vi "readAllSettings.vi"(8 "error in (no error)":errorcluster) -> (0 "error out":errorcluster, 3 "ILC Settings":T1={"Collection Settings"={"Samples To Average"=1, "Test Delay"=0.01}, "TestExecutionOrder"=[], "Verify Voltage Tests"={"+3.3VD"={"DAQ Channel to Read"="ai3", "Expected Value"=0.0, "Tolerance"=0.0}, "+5.1V"={"DAQ Channel to Read"="ai3", "Expected Value"=0.0, "Tolerance"=0.0}, "RELVALV1"={"DAQ Channel to Read"="", "Expected Value"=0.0, "Tolerance"=0.0}, "RELVALV2"={"DAQ Channel to Read"="", "Expected Value"=0.0, "Tolerance"=0.0}}, "Verify DAC Tests"={"DAC A Channels"={"DAQ Channel 1 to Read"="ai5", "DAQ Channel 2 to Read"="ai6", "Resistor Ohms"=0.0}, "DAC B Channels"={"DAQ Channel 1 to Read"="ai7", "DAQ Channel 2 to Read"="ai8", "Resistor Ohms"=0.0}, "DAC = -1.00A"={"Expected Value"=-1.0, "Tolerance"=0.001}, "DAC = -0.75A"={"Expected Value"=-0.75, "Tolerance"=0.00075}, "DAC = -0.50A"={"Expected Value"=-0.5, "Tolerance"=0.0005}, "DAC = -0.25A"={"Expected Value"=-0.25, "Tolerance"=0.00025}, "DAC = 0.00A"={"Expected Value"=0.0, "Tolerance"=0.0001}, "DAC = 0.25A"={"Expected Value"=0.25, "Tolerance"=0.00025}, "DAC = 0.50A"={"Expected Value"=0.5, "Tolerance"=0.0005}, "DAC = 0.75A"={"Expected Value"=0.75, "Tolerance"=0.00075}, "DAC = 1.00A"={"Expected Value"=1.0, "Tolerance"=0.001}}, "Set DAC Tests"={"DAC = 0.00A"={"Command Value"=34224}, "DAC = 0.25A"={"Command Value"=42052}, "DAC = 0.5A"={"Command Value"=49879}, "DAC = 0.75A"={"Command Value"=57707}, "DAC = 1.0A"={"Command Value"=65535}, "DAC = -0.25A"={"Command Value"=26396}, "DAC = -0.5A"={"Command Value"=18568}, "DAC = -0.75A"={"Command Value"=10740}, "DAC = -1.0A"={"Command Value"=0}}, "Enable Disable"={"Motor Enable"=255, "Motor Disable"=0, "Current Output Enable"=1, "Current Output Disable"=0, "Power Enable"=0, "Power Disable"=1, "Amplifier Enable"=0, "Amplifier Disable"=1}, "Pressure Tests"={"0% Test"={"Command"=0, "Expected"=1933, "Tolerance"=492}, "25% Test"={"Command"=12322, "Expected"=4095, "Tolerance"=492}, "50% Test"={"Command"=26326, "Expected"=6553, "Tolerance"=492}, "75% Test"={"Command"=40329, "Expected"=9010, "Tolerance"=492}, "100% Test"={"Command"=54332, "Expected"=11468, "Tolerance"=492}, "Settling (ms)"=500, "Delay (ms)"=10}} {"Verify DAC Tests"."DAC = 1.00A"."Tolerance" format="%.6f"; "Verify DAC Tests"."DAC = 1.00A"."Expected Value" format="%.3f"; "Verify DAC Tests"."DAC = 0.75A"."Tolerance" format="%.6f"; "Verify DAC Tests"."DAC = 0.75A"."Expected Value" format="%.3f"; "Verify DAC Tests"."DAC = 0.50A"."Tolerance" format="%.6f"; "Verify DAC Tests"."DAC = 0.50A"."Expected Value" format="%.3f"; "Verify DAC Tests"."DAC = 0.25A"."Tolerance" format="%.6f"; "Verify DAC Tests"."DAC = 0.25A"."Expected Value" format="%.3f"; "Verify DAC Tests"."DAC = 0.00A"."Tolerance" format="%.6f"; "Verify DAC Tests"."DAC = 0.00A"."Expected Value" format="%.3f"; "Verify DAC Tests"."DAC = -0.25A"."Tolerance" format="%.6f"; "Verify DAC Tests"."DAC = -0.25A"."Expected Value" format="%.3f"; "Verify DAC Tests"."DAC = -0.50A"."Tolerance" format="%.6f"; "Verify DAC Tests"."DAC = -0.50A"."Expected Value" format="%.3f"; "Verify DAC Tests"."DAC = -0.75A"."Tolerance" format="%.6f"; "Verify DAC Tests"."DAC = -0.75A"."Expected Value" format="%.3f"; "Verify DAC Tests"."DAC = -1.00A"."Tolerance" format="%.6f"; "Verify DAC Tests"."DAC = -1.00A"."Expected Value" format="%.3f"; "Verify DAC Tests"."DAC B Channels"."Resistor Ohms" format="%.3g"; "Verify DAC Tests"."DAC A Channels"."Resistor Ohms" format="%.3g"; "Verify Voltage Tests"."RELVALV2"."Tolerance" format="%.6f"; "Verify Voltage Tests"."RELVALV2"."Expected Value" format="%.3f"; "Verify Voltage Tests"."RELVALV1"."Tolerance" format="%.6f"; "Verify Voltage Tests"."RELVALV1"."Expected Value" format="%.3f"; "Verify Voltage Tests"."+5.1V"."Tolerance" format="%.6f"; "Verify Voltage Tests"."+5.1V"."Expected Value" format="%.3f"; "Verify Voltage Tests"."+3.3VD"."Tolerance" format="%.6f"; "Verify Voltage Tests"."+3.3VD"."Expected Value" format="%.3f"})   [LabVIEW 2015]
uses:
  Typedefs/Test Settings.ctl
  Typedefs/Collection Settings.ctl
  Typedefs/TestExecutionOrder.ctl
  Typedefs/TestScenarioTypes.ctl
  Typedefs/Verify Voltage Tests.ctl
  Typedefs/Verify Voltage Test.ctl
  Typedefs/Verify DAC Tests.ctl
  Typedefs/DAC Channels.ctl
  Typedefs/Verify DAC Test.ctl
  Typedefs/Set DAC Tests.ctl
  Typedefs/Set DAC Test.ctl
  Typedefs/Enable Disable.ctl
  Typedefs/Pressure Tests.ctl
  Typedefs/Pressure Test.ctl
  ConfigurationTestParameters/ConfigurationTestParameters.lvclass
  Typedefs/ILCBTTypedefs.lvlib
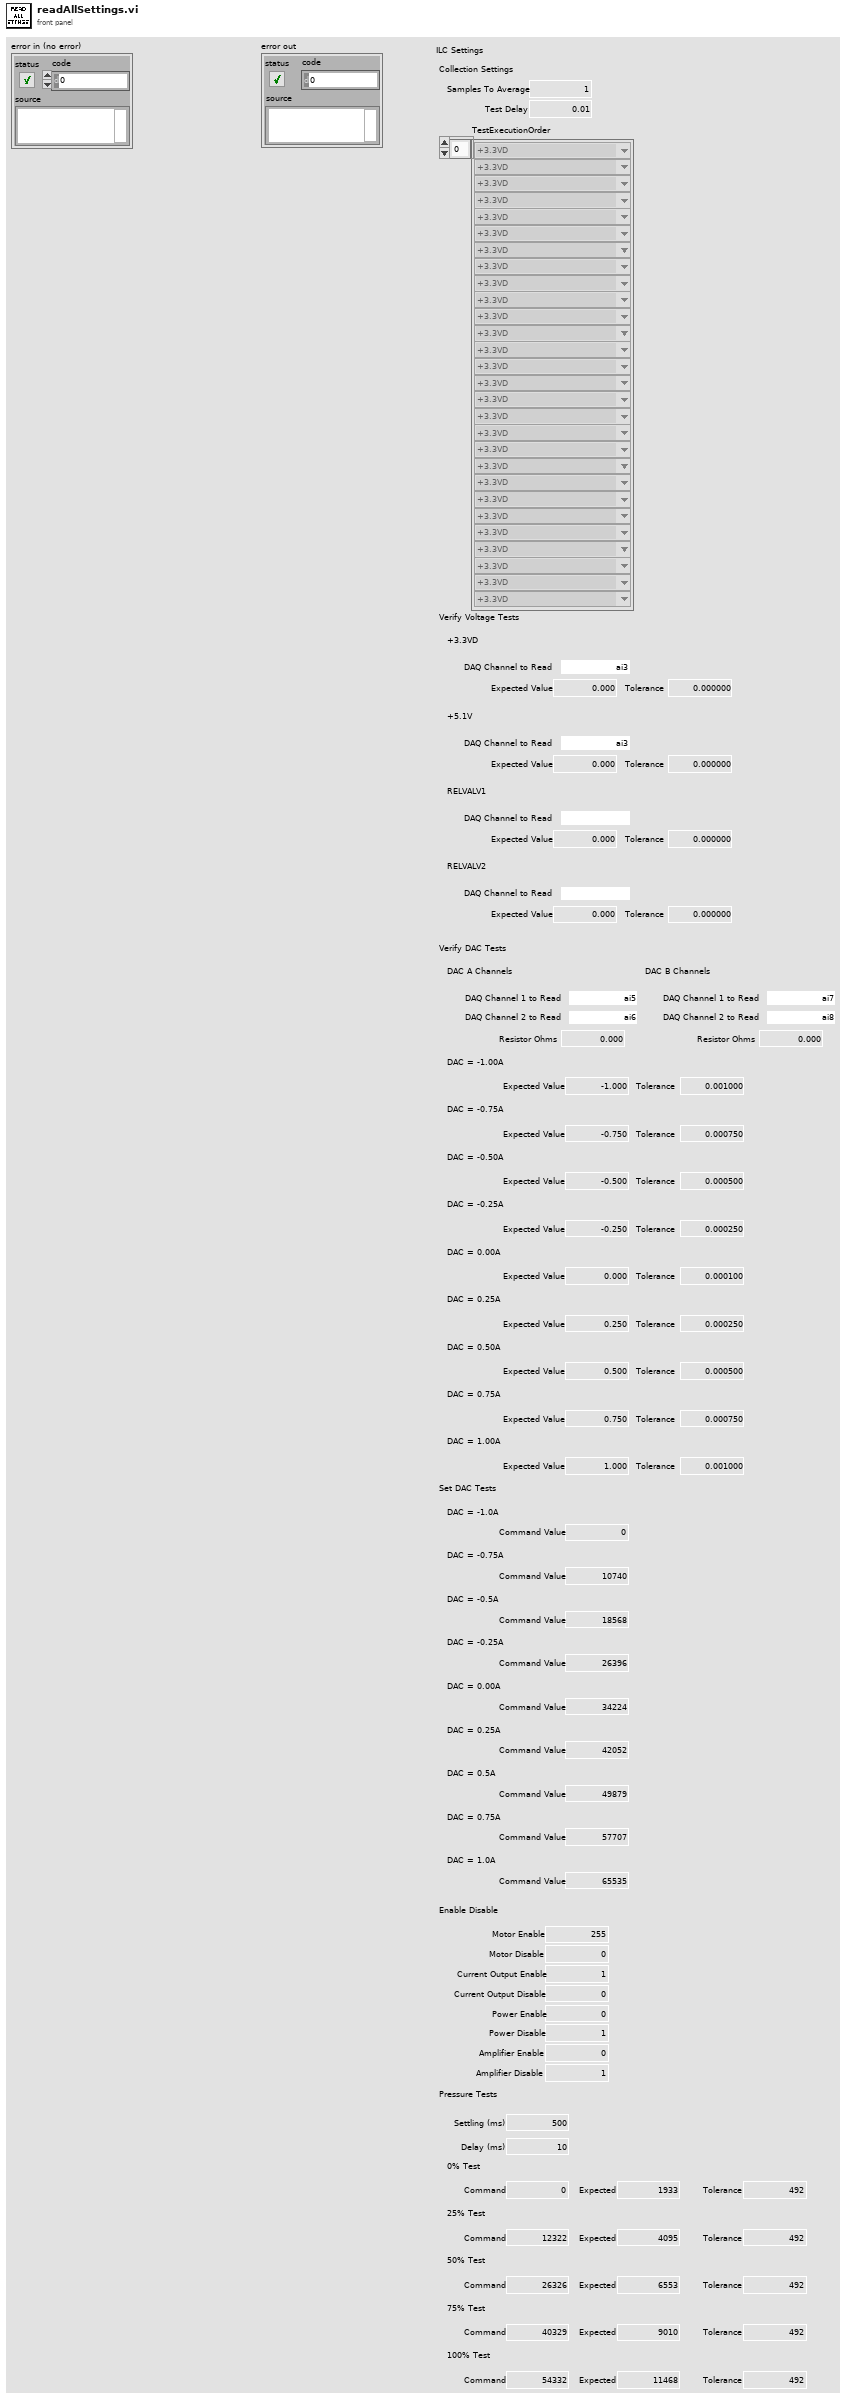
[diagram p1: front panel]
types:
  T1 = typedef "ILCBTTypedefs.lvlib/Test Settings.ctl" = cluster{"Collection Settings":T2, "TestExecutionOrder":T3, "Verify Voltage Tests":T5, "Verify DAC Tests":T7, "Set DAC Tests":T10, "Enable Disable":T12, "Pressure Tests":T13}
  T2 = typedef "ILCBTTypedefs.lvlib/Collection Settings.ctl" = cluster{"Samples To Average":i32, "Test Delay":dbl}
  T3 = typedef "ILCBTTypedefs.lvlib/TestExecutionOrder.ctl" = T4[]
  T4 = typedef "ILCBTTypedefs.lvlib/TestScenarioTypes.ctl" = enum16{"+3.3VD", "+5.1V", "+24V", "RELVALV1", "RELVALV2", "Verify DAC_A = -1.00A", "Verify DAC_A = -0.75A", "Verify DAC_A = -0.50A", "Verify DAC_A = -0.25A", "Verify DAC_A = 0.00A", "Verify DAC_A = 0.25A", "Verify DAC_A = 0.50A", "Verify DAC_A = 0.75A", "Verify DAC_A = 1.00A", "Verify DAC_B = -1.00A", "Verify DAC_B = -0.75A", "Verify DAC_B = -0.50A", "Verify DAC_B = -0.25A", "Verify DAC_B = 0.00A", "Verify DAC_B = 0.25A", "Verify DAC_B = 0.50A", "Verify DAC_B = 0.75A", "Verify DAC_B = 1.00A", "Set DAC_A = -1.00A", "Set DAC_A = -0.75A", "Set DAC_A = -0.50A", "Set DAC_A = -0.25A", "Set DAC_A = 0.00A", "Set DAC_A = 0.25A", "Set DAC_A = 0.50A", "Set DAC_A = 0.75A", "Set DAC_A = 1.00A", "Set DAC_B = -1.00A", "Set DAC_B = -0.75A", "Set DAC_B = -0.50A", "Set DAC_B = -0.25A", "Set DAC_B = 0.00A", "Set DAC_B = 0.25A", "Set DAC_B = 0.50A", "Set DAC_B = 0.75A", "Set DAC_B = 1.00A", "Set MTR_PWR = On", "Set MTR_PWR = Off", "Set OUTPUT = On", "Set OUTPUT = Off", "Verify OUTPUT = On", "Verify OUTPUT = Off", "Verify POWER = Ok", "Verify POWER = Fail", "Verify AMP1 = Ok", "Verify AMP1 = Fail", "Verify AMP2 = Ok", "Verify AMP2 = Fail", "P1 0%", "P1 25%", "P1 50%", "P1 75%", "P1 100%", "P2 0%", "P2 25%", "P2 50%", "P2 75%", "P2 100%", "P3 0%", "P3 25%", "P3 50%", "P3 75%", "P3 100%", "P4 0%", "P4 25%", "P4 50%", "P4 75%", "P4 100%"}
  T5 = typedef "ILCBTTypedefs.lvlib/Verify Voltage Tests.ctl" = cluster{"+3.3VD":T6, "+5.1V":T6, "RELVALV1":T6, "RELVALV2":T6}
  T6 = typedef "ILCBTTypedefs.lvlib/Verify Voltage Test.ctl" = cluster{"DAQ Channel to Read":refnum<k21>, "Expected Value":dbl, "Tolerance":dbl}
  T7 = typedef "ILCBTTypedefs.lvlib/Verify DAC Tests.ctl" = cluster{"DAC A Channels":T8, "DAC B Channels":T8, "DAC = -1.00A":T9, "DAC = -0.75A":T9, "DAC = -0.50A":T9, "DAC = -0.25A":T9, "DAC = 0.00A":T9, "DAC = 0.25A":T9, "DAC = 0.50A":T9, "DAC = 0.75A":T9, "DAC = 1.00A":T9}
  T8 = typedef "ILCBTTypedefs.lvlib/DAC Channels.ctl" = cluster{"DAQ Channel 1 to Read":refnum<k21>, "DAQ Channel 2 to Read":refnum<k21>, "Resistor Ohms":dbl}
  T9 = typedef "ILCBTTypedefs.lvlib/Verify DAC Test.ctl" = cluster{"Expected Value":dbl, "Tolerance":dbl}
  T10 = typedef "ILCBTTypedefs.lvlib/Set DAC Tests.ctl" = cluster{"DAC = 0.00A":T11, "DAC = 0.25A":T11, "DAC = 0.5A":T11, "DAC = 0.75A":T11, "DAC = 1.0A":T11, "DAC = -0.25A":T11, "DAC = -0.5A":T11, "DAC = -0.75A":T11, "DAC = -1.0A":T11}
  T11 = typedef "ILCBTTypedefs.lvlib/Set DAC Test.ctl" = cluster{"Command Value":u16}
  T12 = typedef "ILCBTTypedefs.lvlib/Enable Disable.ctl" = cluster{"Motor Enable":u16, "Motor Disable":u16, "Current Output Enable":u16, "Current Output Disable":u16, "Power Enable":u16, "Power Disable":u16, "Amplifier Enable":u16, "Amplifier Disable":u16}
  T13 = typedef "ILCBTTypedefs.lvlib/Pressure Tests.ctl" = cluster{"0% Test":T14, "25% Test":T14, "50% Test":T14, "75% Test":T14, "100% Test":T14, "Settling (ms)":u16, "Delay (ms)":u16}
  T14 = typedef "ILCBTTypedefs.lvlib/Pressure Test.ctl" = cluster{"Command":u16, "Expected":u16, "Tolerance":u16}
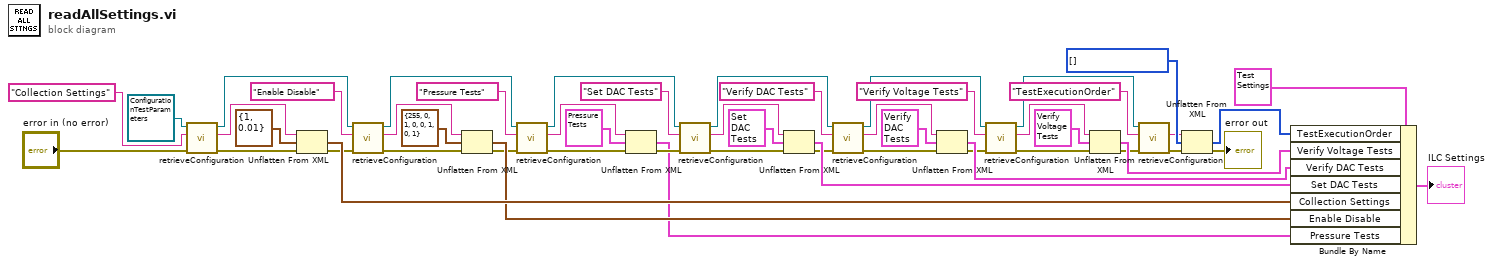
[diagram p0: block diagram]
diagram:
  w24 = T3 [] items=["+3.3VD", "+5.1V", "+24V", "RELVALV1", "RELVALV2", "Verify DAC_A = -1.00A", "Verify DAC_A = -0.75A", "Verify DAC_A = -0.50A", "Verify DAC_A = -0.25A", "Verify DAC_A = 0.00A", "Verify DAC_A = 0.25A", "Verify DAC_A = 0.50A", "Verify DAC_A = 0.75A", "Verify DAC_A = 1.00A", "Verify DAC_B = -1.00A", "Verify DAC_B = -0.75A", "Verify DAC_B = -0.50A", "Verify DAC_B = -0.25A", "Verify DAC_B = 0.00A", "Verify DAC_B = 0.25A", "Verify DAC_B = 0.50A", "Verify DAC_B = 0.75A", "Verify DAC_B = 1.00A", "Set DAC_A = -1.00A", "Set DAC_A = -0.75A", "Set DAC_A = -0.50A", "Set DAC_A = -0.25A", "Set DAC_A = 0.00A", "Set DAC_A = 0.25A", "Set DAC_A = 0.50A", "Set DAC_A = 0.75A", "Set DAC_A = 1.00A", "Set DAC_B = -1.00A", "Set DAC_B = -0.75A", "Set DAC_B = -0.50A", "Set DAC_B = -0.25A", "Set DAC_B = 0.00A", "Set DAC_B = 0.25A", "Set DAC_B = 0.50A", "Set DAC_B = 0.75A", "Set DAC_B = 1.00A", "Set MTR_PWR = On", "Set MTR_PWR = Off", "Set OUTPUT = On", "Set OUTPUT = Off", "Verify OUTPUT = On", "Verify OUTPUT = Off", "Verify POWER = Ok", "Verify POWER = Fail", "Verify AMP1 = Ok", "Verify AMP1 = Fail", "Verify AMP2 = Ok", "Verify AMP2 = Fail", "P1 0%", "P1 25%", "P1 50%", "P1 75%", "P1 100%", "P2 0%", "P2 25%", "P2 50%", "P2 75%", "P2 100%", "P3 0%", "P3 25%", "P3 50%", "P3 75%", "P3 100%", "P4 0%", "P4 25%", "P4 50%", "P4 75%", "P4 100%"] ("TestExecutionOrder")
  n1 = call "retrieveConfiguration.vi"("error in (no error)"="error in (no error)", "configName"="Collection Settings", "ConfigurationThisComponent in"=refnum<class "ConfigurationTestParameters.lvclass"> refnum ("ConfigurationTestParameters.lvclass")) -> ("error out"=w18:errorcluster, "xmlConfig"=w17:string, "ConfigurationThisComponent out"=w16:refnum<class "ConfigurationTestParameters.lvclass">)  [unwired: 6 in]
  n2 = Unflatten From XML(xml string=w17, type=T2 {"Samples To Average"=1, "Test Delay"=0.01} ("Collection Settings"), error in (no error)=w18) -> (value=w52:T2, error out=w15:errorcluster)
  n3 = call "retrieveConfiguration.vi"("error in (no error)"=w15, "configName"="Enable Disable", "ConfigurationThisComponent in"=w16) -> ("error out"=w12:errorcluster, "xmlConfig"=w13:string, "ConfigurationThisComponent out"=w6:refnum<class "ConfigurationTestParameters.lvclass">)  [unwired: 6 in]
  n4 = Unflatten From XML(xml string=w13, type=T12 {"Motor Enable"=255, "Motor Disable"=0, "Current Output Enable"=1, "Current Output Disable"=0, "Power Enable"=0, "Power Disable"=1, "Amplifier Enable"=0, "Amplifier Disable"=1} ("Enable / Disable"), error in (no error)=w12) -> (value=w10:T12, error out=w2:errorcluster)
  n5 = call "retrieveConfiguration.vi"("error in (no error)"=w2, "configName"="Pressure Tests", "ConfigurationThisComponent in"=w6) -> ("error out"=w3:errorcluster, "xmlConfig"=w4:string, "ConfigurationThisComponent out"=w5:refnum<class "ConfigurationTestParameters.lvclass">)  [unwired: 6 in]
  n6 = Unflatten From XML(xml string=w4, type=T13 {"0% Test"={"Command"=0, "Expected"=1933, "Tolerance"=492}, "25% Test"={"Command"=12322, "Expected"=4095, "Tolerance"=492}, "50% Test"={"Command"=26326, "Expected"=6553, "Tolerance"=492}, "75% Test"={"Command"=40329, "Expected"=9010, "Tolerance"=492}, "100% Test"={"Command"=54332, "Expected"=11468, "Tolerance"=492}, "Settling (ms)"=500, "Delay (ms)"=10} ("Pressure Tests"), error in (no error)=w3) -> (value=w7:T13, error out=w8:errorcluster)
  n7 = call "retrieveConfiguration.vi"("error in (no error)"=w8, "configName"="Set DAC Tests", "ConfigurationThisComponent in"=w5) -> ("error out"=w44:errorcluster, "xmlConfig"=w37:string, "ConfigurationThisComponent out"=w30:refnum<class "ConfigurationTestParameters.lvclass">)  [unwired: 6 in]
  n8 = Unflatten From XML(xml string=w37, type=T10 {"DAC = 0.00A"={"Command Value"=34224}, "DAC = 0.25A"={"Command Value"=42052}, "DAC = 0.5A"={"Command Value"=49879}, "DAC = 0.75A"={"Command Value"=57707}, "DAC = 1.0A"={"Command Value"=65535}, "DAC = -0.25A"={"Command Value"=26396}, "DAC = -0.5A"={"Command Value"=18568}, "DAC = -0.75A"={"Command Value"=10740}, "DAC = -1.0A"={"Command Value"=0}} ("Set DAC Tests"), error in (no error)=w44) -> (value=w51:T10, error out=w40:errorcluster)
  n9 = call "retrieveConfiguration.vi"("error in (no error)"=w40, "configName"="Verify DAC Tests", "ConfigurationThisComponent in"=w30) -> ("error out"=w43:errorcluster, "xmlConfig"=w38:string, "ConfigurationThisComponent out"=w31:refnum<class "ConfigurationTestParameters.lvclass">)  [unwired: 6 in]
  n10 = Unflatten From XML(xml string=w38, type=T7 {"DAC A Channels"={"DAQ Channel 1 to Read"="", "DAQ Channel 2 to Read"="ai6", "Resistor Ohms"=0.0}, "DAC B Channels"={"DAQ Channel 1 to Read"="ai7", "DAQ Channel 2 to Read"="ai8", "Resistor Ohms"=0.0}, "DAC = -1.00A"={"Expected Value"=-1.0, "Tolerance"=0.001}, "DAC = -0.75A"={"Expected Value"=-0.75, "Tolerance"=0.00075}, "DAC = -0.50A"={"Expected Value"=-0.5, "Tolerance"=0.0005}, "DAC = -0.25A"={"Expected Value"=-0.25, "Tolerance"=0.00025}, "DAC = 0.00A"={"Expected Value"=0.0, "Tolerance"=0.0001}, "DAC = 0.25A"={"Expected Value"=0.25, "Tolerance"=0.00025}, "DAC = 0.50A"={"Expected Value"=0.5, "Tolerance"=0.0005}, "DAC = 0.75A"={"Expected Value"=0.75, "Tolerance"=0.00075}, "DAC = 1.00A"={"Expected Value"=1.0, "Tolerance"=0.001}} ("Verify DAC Tests"), error in (no error)=w43) -> (value=w50:T7, error out=w41:errorcluster)
  n11 = call "retrieveConfiguration.vi"("error in (no error)"=w41, "configName"="Verify Voltage Tests", "ConfigurationThisComponent in"=w31) -> ("error out"=w42:errorcluster, "xmlConfig"=w39:string, "ConfigurationThisComponent out"=w21:refnum<class "ConfigurationTestParameters.lvclass">)  [unwired: 6 in]
  n12 = Unflatten From XML(xml string=w39, type=T5 {"+3.3VD"={"DAQ Channel to Read"="ai3", "Expected Value"=3.3, "Tolerance"=0.0}, "+5.1V"={"DAQ Channel to Read"="ai3", "Expected Value"=5.1, "Tolerance"=0.0}, "RELVALV1"={"DAQ Channel to Read"="ai3", "Expected Value"=2.4, "Tolerance"=0.0024}, "RELVALV2"={"DAQ Channel to Read"="ai4", "Expected Value"=2.4, "Tolerance"=0.0024}} ("Verify Voltage Tests"), error in (no error)=w42) -> (value=w49:T5, error out=w27:errorcluster)
  n13 = call "retrieveConfiguration.vi"("error in (no error)"=w27, "configName"="TestExecutionOrder", "ConfigurationThisComponent in"=w21) -> ("error out"=w26:errorcluster, "xmlConfig"=w23:string)  [unwired: 6 in, 1 out]
  n14 = Unflatten From XML(xml string=w23, type=w24, error in (no error)=w26) -> (value=w22:T3, error out=→"error out":errorcluster)
  n15 = Bundle By Name(cluster=T1 {"Collection Settings"={"Samples To Average"=1, "Test Delay"=0.01}, "TestExecutionOrder"=[], "Verify Voltage Tests"={"+3.3VD"={"DAQ Channel to Read"="ai3", "Expected Value"=0.0, "Tolerance"=0.0}, "+5.1V"={"DAQ Channel to Read"="ai3", "Expected Value"=0.0, "Tolerance"=0.0}, "RELVALV1"={"DAQ Channel to Read"="", "Expected Value"=0.0, "Tolerance"=0.0}, "RELVALV2"={"DAQ Channel to Read"="", "Expected Value"=0.0, "Tolerance"=0.0}}, "Verify DAC Tests"={"DAC A Channels"={"DAQ Channel 1 to Read"="ai5", "DAQ Channel 2 to Read"="ai6", "Resistor Ohms"=0.0}, "DAC B Channels"={"DAQ Channel 1 to Read"="ai7", "DAQ Channel 2 to Read"="ai8", "Resistor Ohms"=0.0}, "DAC = -1.00A"={"Expected Value"=-1.0, "Tolerance"=0.001}, "DAC = -0.75A"={"Expected Value"=-0.75, "Tolerance"=0.00075}, "DAC = -0.50A"={"Expected Value"=-0.5, "Tolerance"=0.0005}, "DAC = -0.25A"={"Expected Value"=-0.25, "Tolerance"=0.00025}, "DAC = 0.00A"={"Expected Value"=0.0, "Tolerance"=0.0001}, "DAC = 0.25A"={"Expected Value"=0.25, "Tolerance"=0.00025}, "DAC = 0.50A"={"Expected Value"=0.5, "Tolerance"=0.0005}, "DAC = 0.75A"={"Expected Value"=0.75, "Tolerance"=0.00075}, "DAC = 1.00A"={"Expected Value"=1.0, "Tolerance"=0.001}}, "Set DAC Tests"={"DAC = 0.00A"={"Command Value"=34224}, "DAC = 0.25A"={"Command Value"=42052}, "DAC = 0.5A"={"Command Value"=49879}, "DAC = 0.75A"={"Command Value"=57707}, "DAC = 1.0A"={"Command Value"=65535}, "DAC = -0.25A"={"Command Value"=26396}, "DAC = -0.5A"={"Command Value"=18568}, "DAC = -0.75A"={"Command Value"=10740}, "DAC = -1.0A"={"Command Value"=0}}, "Enable Disable"={"Motor Enable"=255, "Motor Disable"=0, "Current Output Enable"=1, "Current Output Disable"=0, "Power Enable"=0, "Power Disable"=1, "Amplifier Enable"=0, "Amplifier Disable"=1}, "Pressure Tests"={"0% Test"={"Command"=0, "Expected"=1933, "Tolerance"=492}, "25% Test"={"Command"=12322, "Expected"=4095, "Tolerance"=492}, "50% Test"={"Command"=26326, "Expected"=6553, "Tolerance"=492}, "75% Test"={"Command"=40329, "Expected"=9010, "Tolerance"=492}, "100% Test"={"Command"=54332, "Expected"=11468, "Tolerance"=492}, "Settling (ms)"=500, "Delay (ms)"=10}} ("ILC Settings"), "TestExecutionOrder"=w22, "Verify Voltage Tests"=w49, "Verify DAC Tests"=w50, "Set DAC Tests"=w51, "Collection Settings"=w52, "Enable Disable"=w10, "Pressure Tests"=w7) -> (→"ILC Settings":T1)
